vi "Untitled 2 (SubVI).vi"(6 "Bool Refnum 4":refnum<vi>, 7 "wybor wykresu in":T1, 8 "error in (no error)":errorcluster, 9 "Bool Refnum 3":refnum<vi>, 10 "Bool Refnum in":refnum<vi>, 11 "Boolean in":refnum<vi>) -> (0 "error out":errorcluster, 3 "wybor wykresu out":T1)   [LabVIEW 2017]
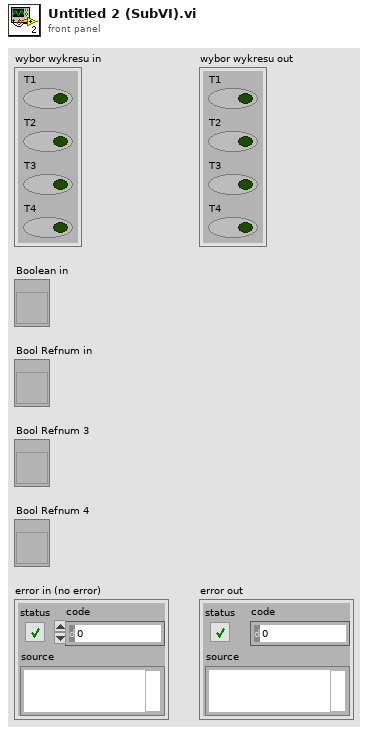
[diagram p1: front panel]
types:
  T1 = cluster{"T1":bool, "T2":bool, "T3":bool, "T4":bool}
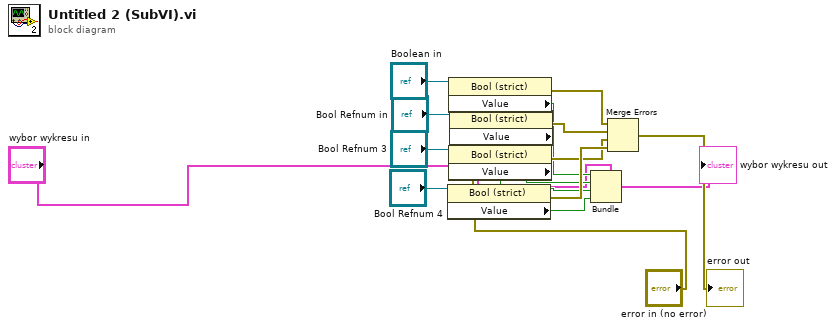
[diagram p0: block diagram]
diagram:
  n1 = property on="Property Node" class="Bool (strict)"(reference="Bool Refnum 4", error in="error in (no error)") -> (error out=w15:errorcluster, "Value"=w9:bool)  [unwired: 1 out]
  n2 = property on="Property Node" class="Bool (strict)"(reference="Boolean in", error in="error in (no error)") -> (error out=w12:errorcluster, "Value"=w6:bool)  [unwired: 1 out]
  n3 = property on="Property Node" class="Bool (strict)"(reference="Bool Refnum 3", error in="error in (no error)") -> (error out=w14:errorcluster, "Value"=w8:bool)  [unwired: 1 out]
  n4 = property on="Property Node" class="Bool (strict)"(reference="Bool Refnum in", error in="error in (no error)") -> (error out=w13:errorcluster, "Value"=w7:bool)  [unwired: 1 out]
  n5 = Bundle(cluster="wybor wykresu in", "T1"=w6, "T2"=w7, "T3"=w8, "T4"=w9) -> (→"wybor wykresu out":T1)
  n6 = Merge Errors(w12, w13, w14, w15) -> (→"error out":errorcluster)
